vi "Cleanup.vi"(8 "error in (no error)":errorcluster, 11 "SequenceViewPanel in":refnum<class "SequenceViewPanel.lvclass">) -> (0 "error out":errorcluster)   [LabVIEW 2020, in "TSnax UI.lvlib" / "SequenceViewPanel.lvclass"]
uses:
  SequenceViewPanel.lvclass
  SequenceViewPanel.lvclass/SequenceViewPanel.ctl
  <vilib>/IlluminatedG/IG OOPanel/OOPanel/Panel/Panel.lvclass
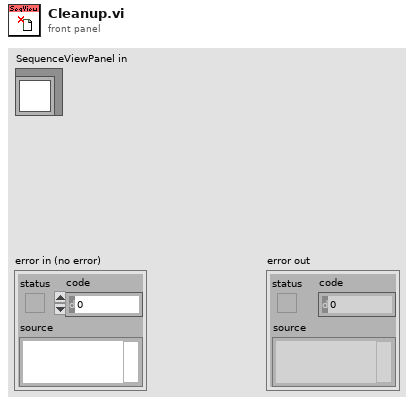
[diagram p1: front panel]
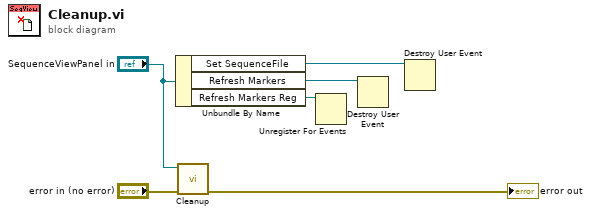
[diagram p0: block diagram]
diagram:
  n1 = Unbundle By Name("SequenceViewPanel in") -> ("Set SequenceFile"=w6:refnum<user-event>, "Refresh Markers"=w1:refnum<user-event>, "Refresh Markers Reg"=w2:refnum<event-registration>)
  n2 = call-parent "Cleanup.vi"("error in (no error)"="error in (no error)", "Panel in"="SequenceViewPanel in") -> ("error out"=→"error out":errorcluster)  [unwired: 9 in]
  n3 = Unregister For Events(event registration refnum=w2) -> ()  [unwired: 1 in, 1 out]
  n4 = Destroy User Event(user event=w1) -> ()  [unwired: 1 in, 1 out]
  n5 = Destroy User Event(user event=w6) -> ()  [unwired: 1 in, 1 out]
